vi "EnFlo_Tun_Setup_global.vi"() -> ()   [LabVIEW 2010]
panel:
  in  "Aero Tunnel DB array":string[][](array[string])
  in  "D Tunnel DB array":string[][](array[string])
  in  "A Tunnel DB array":string[][](array[string])
  in  "EnFlo Tun DB array":string[][](array[string])
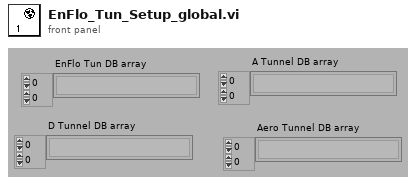
[diagram p1: front panel]
diagram:
